vi "midiInReset.vi"(8 "error in":errorcluster, 11 "midi in":refnum<class "midi.lvclass">) -> (0 "error out":errorcluster, 3 "midi out":refnum<class "midi.lvclass">)   [LabVIEW 2020, in "midi.lvclass"]
doc: "The midiInReset function stops input on a given MIDI input device.\n\nThis function returns all pending input buffers to the callback function and sets the MHDR_DONE flag in the dwFlags member of the MIDIHDR structure."
uses:
  midi.lvclass
  midi.lvclass/midi.ctl
  winmm.dll
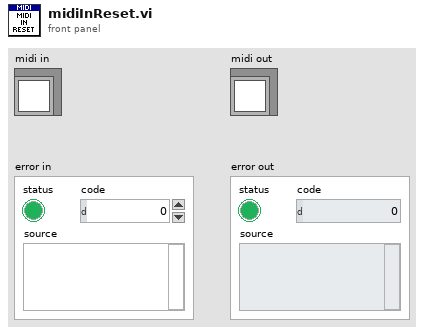
[diagram p1: front panel]
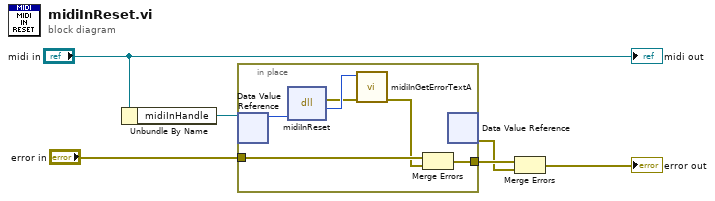
[diagram p0: block diagram]
diagram:
  n1 = Unbundle By Name("midi in") -> ("midiInHandle"=w4:refnum<data-value>)
  n2 = in-place {
    in-place-border: "error in" -> [w10]
    in-place-border: [w8] -> w3
    n3 = in-place-dvr #1(w4) -> (w7:u64)  [unwired: 1 out]
    n4 = dll-call lib="winmm.dll" fn="midiInReset"("hmi"=w7) -> (error out=w11:errorcluster, "return type"=w12:i32)  [unwired: 4 in, 1 out]
    n5 = call "midiInGetErrorTextA.vi"("error in"=w11, "Error Code"=w12) -> ("error out"=w9:errorcluster)  [unwired: 9 in]
    n6 = Merge Errors(w10, w9) -> (w8:errorcluster)
    n7 = in-place-dvr #1() -> (w2:errorcluster)  [unwired: 1 in, 1 out]
  }
  n8 = Merge Errors(w3, w2) -> (→"error out":errorcluster)
  "midi out" <- "midi in"
